vi "I2C LCD Full.vi"() -> ()   [LabVIEW 2020, in "CTI-Scratchpad.lvlib"]
uses:
  CTI-Scratchpad.lvlib
  CTI/VisaComms/VisaComms.lvclass
  CTI-Peripheral/Grove I2C LCD/Grove I2C LCD.lvclass
  CTI/Session/Session.lvclass
  CTI-Peripheral/PCF8574 I2C LCD/PCF8574 I2C LCD.lvclass
  CTI-Peripheral/Character LCD/Char LCD.lvclass
  C:/dev/cti/cti-drivers-lv-visa/CTI-Peripheral/Grove I2C LCD/Grove I2C LCD.lvclass
  C:/dev/cti/cti-drivers-lv-visa/CTI-Peripheral/Character LCD/Char LCD.lvclass
  C:/dev/cti/cti-drivers-lv-visa/CTI-Peripheral/PCF8574 I2C LCD/PCF8574 I2C LCD.lvclass
  CTI-Visa-DeviceLib/LCD-I2C/Position.ctl
  CTI-Visa-DeviceLib/LCD-I2C/Custom Char.ctl
  CTI/I2C Number.ctl
  CTI/CTI.lvlib
  CTI/GPIO Number.ctl
  CTI/I2C Address.ctl
  CTI/Identity.ctl
panel:
  out "Identity":T1
  in  "LCD Type":enum32{"Grove", "PCF8574"}(tab)
  in  "Address":T2=39 format="%02x"
  in  "SDA GPIO":T3=8
  in  "SCL GPIO":T3=9
  in  "Baud":u32=400000 format="%.0p"
  in  "I2C #":T4
  in  "Custom Chars":T6
  in  "Backlight":bool=TRUE
  in  "Create":bool
  in  "stop":bool
  out "error out":errorcluster
  in  "Scroll Right":bool
  in  "Scroll Left":bool
  in  "Home":bool
  in  "Clear":bool
  in  "Write Text":bool
  in  "Text":string="Hello LabVIEW!"
  in  "Port":refnum<visa-resource-name>="COM5"
  in  "Goto":bool
  in  "Position":T7
  in  "Display":bool=TRUE
  in  "Blink":bool
  in  "Cursor":bool=TRUE
  # "Use \\00 through \\07 to specify custom chars"
  # "No additional\nConfig"
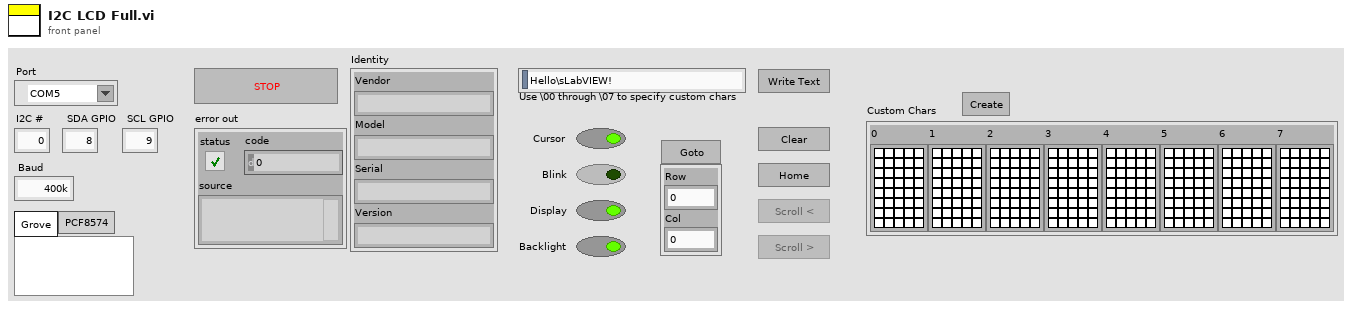
[diagram p1: front panel]
types:
  T1 = typedef "CTI.lvlib/Identity.ctl" = cluster{"Vendor":string, "Model":string, "Serial":string, "Version":string}
  T2 = typedef "CTI.lvlib/I2C Address.ctl" = u8
  T3 = typedef "CTI.lvlib/GPIO Number.ctl" = i8
  T4 = typedef "CTI.lvlib/I2C Number.ctl" = i8
  T5 = typedef "CTI-Visa-DeviceLib.lvlib/LCD-I2C.lvclass/Custom Char.ctl" = bool[][]
  T6 = cluster{"0":T5, "1":T5, "2":T5, "3":T5, "4":T5, "5":T5, "6":T5, "7":T5}
  T7 = typedef "CTI-Visa-DeviceLib.lvlib/LCD-I2C.lvclass/Position.ctl" = cluster{"Row":u8, "Col":u8}
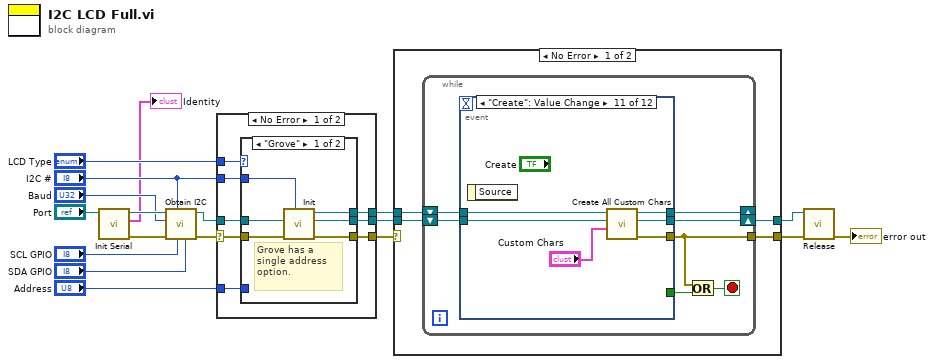
[diagram p0: block diagram]
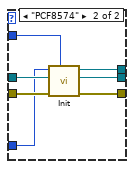
[diagram p2: hidden frame]
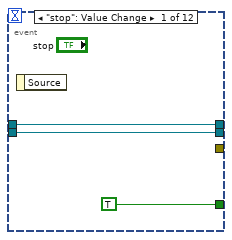
[diagram p4: hidden frame]
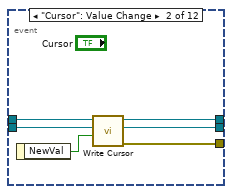
[diagram p5: hidden frame]
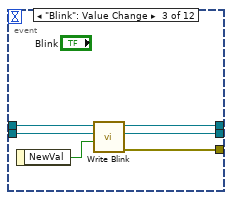
[diagram p6: hidden frame]
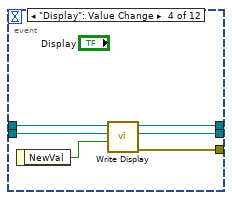
[diagram p7: hidden frame]
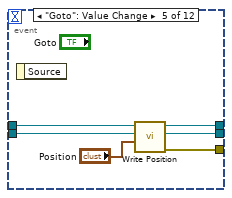
[diagram p8: hidden frame]
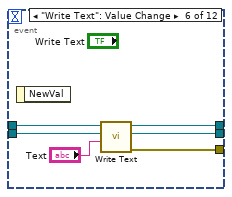
[diagram p9: hidden frame]
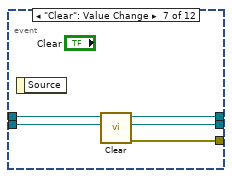
[diagram p10: hidden frame]
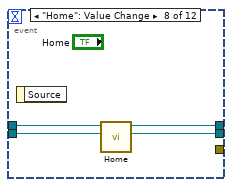
[diagram p11: hidden frame]
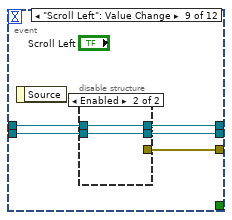
[diagram p12: hidden frame]
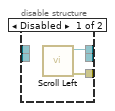
[diagram p13: hidden frame]
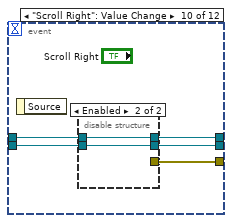
[diagram p14: hidden frame]
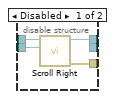
[diagram p15: hidden frame]
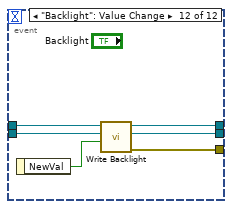
[diagram p16: hidden frame]
diagram:
  n1 = call "Init Serial.vi"("VISA resource name in"="Port") -> ("error out"=w17:errorcluster, "Identity"=→"Identity":T1, "Session"=w9:refnum<class "Session.lvclass">)  [unwired: 8 in]
  n2 = call "Obtain I2C.vi"("SDA GPIO"="SDA GPIO", "SCL GPIO"="SCL GPIO", "I2C #"="I2C #", "error in (no error)"=w17, "Baud"="Baud", "Session in"=w9) -> ("error out"=w10:errorcluster, "Session out"=w8:refnum<class "Session.lvclass">)  [unwired: 4 in]
  n3 = case shown="No Error" w10 {
    selector: w10 -> [w23 w41]
    tunnel: [w26 w41] -> w16
    tunnel: [w25 w40] -> w15
    tunnel: [w24 _] -> w14
    tunnel: w8 -> [w22 w40]
    tunnel: "I2C #" -> [w21 _]
    tunnel: "LCD Type" -> [w20 _]
    tunnel: "Address" -> [w19 _]
    frame No Error {
      n4 = case shown="\"Grove\"" w20 {
        tunnel: [w32 w38] -> w26
        tunnel: [w31 w37] -> w25
        tunnel: [w30 w36] -> w24
        tunnel: w23 -> [w29 w39]
        tunnel: w22 -> [w28 w34]
        tunnel: w21 -> [w27 w35]
        tunnel: w19 -> [_ w33]
        frame "Grove" {
          # "Grove has a single address option."
          n5 = call "Init.vi"("I2C #"=w27, "error in (no error)"=w29, "Session In"=w28) -> ("error out"=w32:errorcluster, "Session Out"=w31:refnum<class "Session.lvclass">, "Grove I2C LCD out"=w30:refnum<class "Grove I2C LCD.lvclass">)  [unwired: 6 in]
        }
        frame "PCF8574" {
          n6 = call "Init.vi"("I2C #"=w35, "error in (no error)"=w39, "Session In"=w34, "Address"=w33) -> ("error out"=w38:errorcluster, "Session Out"=w37:refnum<class "Session.lvclass">, "PCF8574 I2C LCD out"=w36:refnum<class "PCF8574 I2C LCD.lvclass">)  [unwired: 5 in]
        }
      }
    }
    frame Error {
    }
  }
  n7 = case shown="No Error" w16 {
    selector: w16 -> [_ w127]
    tunnel: w15 -> [w45 w128]
    tunnel: w14 -> [w44 _]
    tunnel: [w43 w128] -> w13
    tunnel: [w42 w127] -> w12
    frame No Error {
      n8 = while {
        shift-right: [w46] -> _
        shift-left: w44 -> [w52]
        shift-right: [w50] -> w43
        shift-left: w45 -> [w51]
        tunnel: [w47] -> w42
        stop <- w48 stop-if-true
        n9 = event shown="[10] \"Create\": Value Change" {
          selector: _ -> [_ _ _ _ _ _ _ _ _ _ _ _]
          dyn-events: _ -> [_ _ _ _ _ _ _ _ _ _ _ _]
          timeout: _ -> [_ _ _ _ _ _ _ _ _ _ _ _]
          tunnel: w52 -> [w55 w58 w64 w70 w76 w82 w88 w93 w97 w106 w116 w123]
          tunnel: w51 -> [w54 w57 w63 w69 w75 w81 w87 w92 w95 w105 w115 w122]
          tunnel: [w55 w61 w67 w73 w77 w84 w90 w94 w99 w108 w120 w126] -> w46
          tunnel: [w54 w56 w62 w68 w74 w80 w86 w91 w96 w104 w117 w121] -> w50
          tunnel: [TRUE _ _ _ _ _ _ _ _ _ _ _] -> w49
          tunnel: [_ w59 w65 w71 w78 w83 w89 _ w98 w107 w119 w124] -> w47
          event "stop": Value Change {
            n10 = event-data() -> ()  [unwired: 1 in, 1 out]
          }
          event "Cursor": Value Change {
            n11 = event-data() -> ("NewVal"=w60:bool)  [unwired: 1 in]
            n12 = call-dynamic "Write Cursor.vi"("Cursor On"=w60, "Session In"=w57, "Char LCD I in"=w58) -> ("error out"=w59:errorcluster, "Session Out"=w56:refnum<class "Session.lvclass">, "Char LCD I out"=w61:refnum<class "Char LCD.lvclass">)  [unwired: 6 in]
          }
          event "Blink": Value Change {
            n13 = event-data() -> ("NewVal"=w66:bool)  [unwired: 1 in]
            n14 = call-dynamic "Write Blink.vi"("Blink On"=w66, "Session In"=w63, "Char LCD I in"=w64) -> ("error out"=w65:errorcluster, "Session Out"=w62:refnum<class "Session.lvclass">, "Char LCD I out"=w67:refnum<class "Char LCD.lvclass">)  [unwired: 6 in]
          }
          event "Display": Value Change {
            n15 = event-data() -> ("NewVal"=w72:bool)  [unwired: 1 in]
            n16 = call-dynamic "Write Display.vi"("Display On"=w72, "Session In"=w69, "Char LCD I in"=w70) -> ("error out"=w71:errorcluster, "Session Out"=w68:refnum<class "Session.lvclass">, "Char LCD I out"=w73:refnum<class "Char LCD.lvclass">)  [unwired: 6 in]
          }
          event "Goto": Value Change {
            n17 = event-data() -> ()  [unwired: 1 in, 1 out]
            n18 = call-dynamic "Write Position.vi"("Position"="Position", "Session In"=w75, "Char LCD I in"=w76) -> ("error out"=w78:errorcluster, "Session Out"=w74:refnum<class "Session.lvclass">, "Char LCD I out"=w77:refnum<class "Char LCD.lvclass">)  [unwired: 6 in]
          }
          event "Write Text": Value Change {
            n19 = event-data() -> ()  [unwired: 1 in, 1 out]
            n20 = call-dynamic "Write Text.vi"("Text"="Text", "Session In"=w81, "Character LCD in"=w82) -> ("error out"=w83:errorcluster, "Session Out"=w80:refnum<class "Session.lvclass">, "Character LCD out"=w84:refnum<class "Char LCD.lvclass">)  [unwired: 6 in]
          }
          event "Clear": Value Change {
            n21 = event-data() -> ()  [unwired: 1 in, 1 out]
            n22 = call-dynamic "Clear.vi"("Session In"=w87, "Character LCD in"=w88) -> ("error out"=w89:errorcluster, "Session Out"=w86:refnum<class "Session.lvclass">, "Character LCD out"=w90:refnum<class "Char LCD.lvclass">)  [unwired: 7 in]
          }
          event "Home": Value Change {
            n23 = event-data() -> ()  [unwired: 1 in, 1 out]
            n24 = call-dynamic "Home.vi"("Session In"=w92, "Character LCD in"=w93) -> ("Session Out"=w91:refnum<class "Session.lvclass">, "Character LCD out"=w94:refnum<class "Char LCD.lvclass">)  [unwired: 7 in, 1 out]
          }
          event "Scroll Left": Value Change {
            n25 = event-data() -> ()  [unwired: 1 in, 1 out]
            n26 = disable-structure shown="Enabled" {
              disable-tunnel: [w101 w103] -> w99
              disable-tunnel: [w100 _] -> w98
              disable-tunnel: w97 -> [_ w103]
              disable-tunnel: [_ w102] -> w96
              disable-tunnel: w95 -> [_ w102]
              frame Disabled {
                n27 = call "Scroll Left.vi"() -> ("error out"=w100:errorcluster, "LCD-I2C out"=w101:refnum<class "LCD-I2C.lvclass">)  [unwired: 9 in, 1 out]
              }
              frame Enabled {
              }
            }
          }
          event "Scroll Right": Value Change {
            n28 = event-data() -> ()  [unwired: 1 in, 1 out]
            n29 = disable-structure shown="Enabled" {
              disable-tunnel: [w112 w113] -> w108
              disable-tunnel: [w111 _] -> w107
              disable-tunnel: w106 -> [w110 w113]
              disable-tunnel: w105 -> [w109 w114]
              disable-tunnel: [_ w114] -> w104
              frame Disabled {
                n30 = call "Scroll Right.vi"("VISA resource name in"=w109, "LCD-I2C in"=w110) -> ("error out"=w111:errorcluster, "LCD-I2C out"=w112:refnum<class "LCD-I2C.lvclass">)  [unwired: 7 in, 1 out]
              }
              frame Enabled {
              }
            }
          }
          event "Create": Value Change {
            n31 = event-data() -> ()  [unwired: 1 in, 1 out]
            n32 = call "Create All Custom Chars.vi"("Custom Chars"="Custom Chars", "Session In"=w115, "Char LCD in"=w116) -> ("error out"=w119:errorcluster, "Session Out"=w117:refnum<class "Session.lvclass">, "Char LCD out"=w120:refnum<class "Char LCD.lvclass">)  [unwired: 6 in]
          }
          event "Backlight": Value Change {
            n33 = event-data() -> ("NewVal"=w125:bool)  [unwired: 1 in]
            n34 = call-dynamic "Write Backlight.vi"("Backlight On"=w125, "Session In"=w122, "Char LCD I in"=w123) -> ("error out"=w124:errorcluster, "Session Out"=w121:refnum<class "Session.lvclass">, "Char LCD I out"=w126:refnum<class "Char LCD.lvclass">)  [unwired: 6 in]
          }
        }
        n35 = Or(x=w47, y=w49) -> (x .or. y?=w48:bool)
      }
    }
    frame Error {
    }
  }
  n36 = call-dynamic "Release.vi"("error in (no error)"=w12, "Session in"=w13) -> ("error out"=→"error out":errorcluster)  [unwired: 9 in]
